vi "Test ToFrom JSONpath Array.vi"() -> ()   [LabVIEW 2017]
uses:
  ba2f4a93-abdc-4bc2-b622-957b07094ab4.vi
  Variant to JSON Text.vi
  JSONtext.lvlib
panel:
  out "error out":errorcluster
  out "<JSON> 2":string
  out "$Paths":string[](array[string])
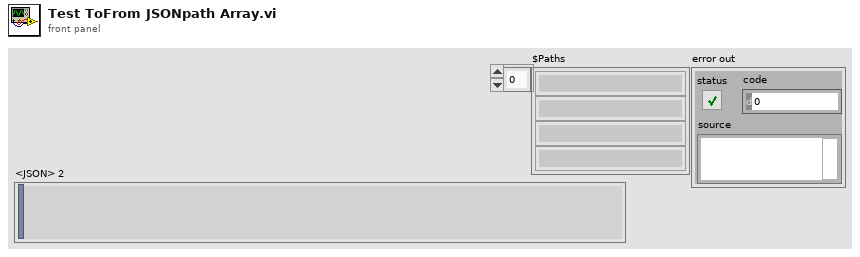
[diagram p1: front panel]
types:
  T1 = cluster{"A0":cluster{"B1":i32, "B2":cluster{"C1":i32, "C2":string}}, "A1":i32, "A2":string, "A3":cluster{"B":cluster{"C":i32[]}}}
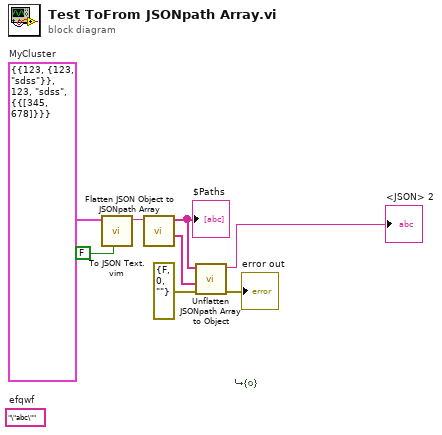
[diagram p0: block diagram]
diagram:
  (unwired) "\"abc\""  # efqwf
  w8 = T1 {"A0"={"B1"=123, "B2"={"C1"=123, "C2"="sdss"}}, "A1"=123, "A2"="sdss", "A3"={"B"={"C"=[345, 678]}}}  # MyCluster
  n1 = call "To JSON Text.vim"("Pretty Print?"=FALSE, "Anything"=w8) -> ("<JSON>"=w6:string)  [unwired: 8 in, 1 out]
  n2 = call "Flatten JSON Object to JSONpath Array.vi"("<JSON> in"=w6) -> ("<JSON>Items"=w1:string[], "$Paths"=w5:string[])  [unwired: 9 in]
  "$Paths" <- w5
  n3 = call "Unflatten JSONpath Array to Object.vi"("error in (no error)"=errorcluster {"status"=FALSE, "code"=0, "source"=""} ("error out"), "<JSON>Items"=w1, "$Paths"=w5) -> ("error out"=→"error out":errorcluster, "<JSON>"=→"<JSON> 2":string)  [unwired: 7 in]
